vi "Averaged_Rot_Measure_Main_v1 Ś kopia.vi"() -> ()   [LabVIEW 2021]
uses:
  Config_File_Paths.ctl
  ZI_Data.ctl
  <vilib>/Utility/file.llb/Write Delimited Spreadsheet (DBL).vi
  <vilib>/measure/maspectr.llb/FFT Spectrum (Real-Im) for 1 Chan.vi
  <vilib>/Analysis/NI_AALPro.lvlib
  <vilib>/measure/NI_MAPro.lvlib
panel:
  out "single spectrum 2":waveform(dbl)[](graph)
  out "averaged spectrum":waveform(dbl)[](graph)
  out "single spectrum":waveform(dbl)[](graph)
  out "single differ":cluster{"Time":dbl[], "X":dbl[]}[](graph)
  out "single abs":cluster{"Time":dbl[], "X":dbl[]}[](graph)
  out "averaged rot":cluster{"Time":dbl[], "X":dbl[]}[](graph)
  out "single rot":cluster{"Time":dbl[], "X":dbl[]}[](graph)
  in  "Resource Address":T1={"ZI Address"="DEV714", "VISA Keithley"="", "VISA Arduino PG"=""}
  in  "error in":errorcluster
  in  "Config files paths":T2={"ZI config file (.ini)"="Config_Ver_1\\Zurich_params.ini", "Keithley config file (.ini)"="Config_Ver_1\\Keithley_params.ini", "Arduino config file (.ini)"="Config_Ver_1\\pulse_sequence.ini"}
  in  "Time unit":string(combo)="ms"
  out "loading":dbl(slide) scale=0.0..100.0
  in  "Number of averages":i32=1
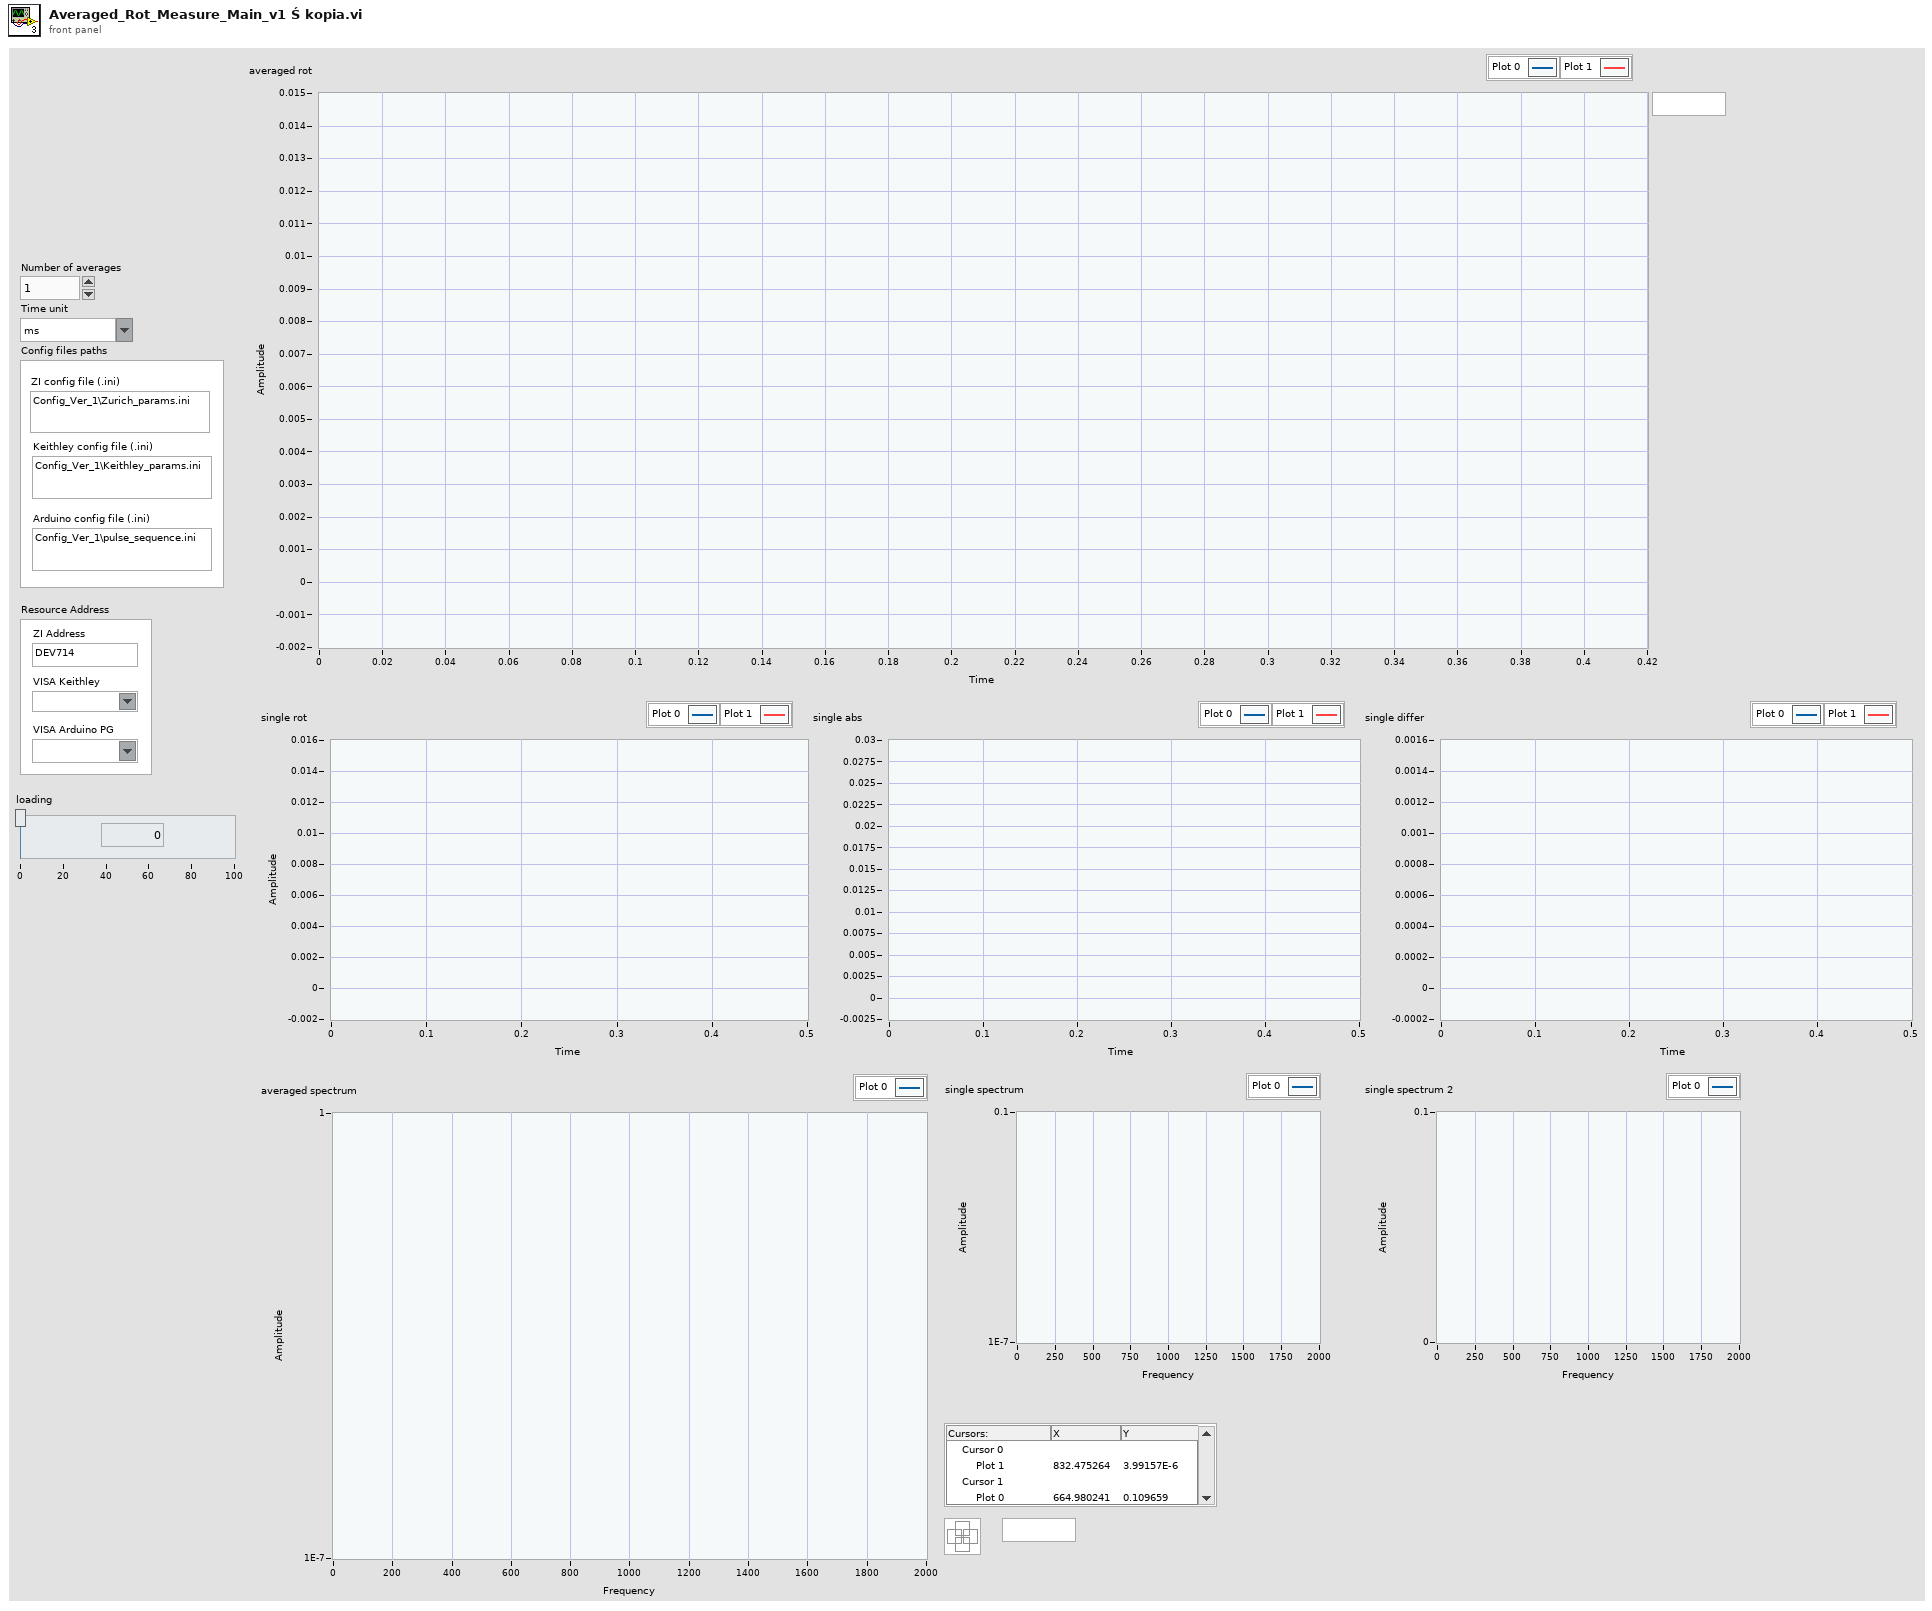
[diagram p1: front panel]
types:
  T1 = cluster{"ZI Address":string, "VISA Keithley":refnum<visa-resource-name>, "VISA Arduino PG":refnum<visa-resource-name>}
  T2 = typedef "Config_File_Paths.ctl" = cluster{"ZI config file (.ini)":string, "Keithley config file (.ini)":string, "Arduino config file (.ini)":string}
  T3 = typedef "ZI_Data.ctl" = cluster{"R":dbl[], "Theta":dbl[], "X":dbl[], "Y":dbl[], "AuxIn0":dbl[], "AuxIn1":dbl[], "Frequency":dbl[], "DIO":dbl[], "Time":dbl[]}
  T4 = typedef "Resources.ctl" = cluster{"ZI Handle":T5, "ZI ModHandle":T6, "VISA arduino":refnum<visa-resource-name>, "VISA Keithley":refnum<visa-resource-name>}
  T5 = typedef "Zurich Instruments LabOne.lvlib/ziTypeHandle.ctl" = cluster{"handleValid":bool, "Conn":u64, "Path Prefix":string, "Handle":u64, "Connected":bool, "Clockbase(s)":dbl}
  T6 = typedef "Zurich Instruments LabOne.lvlib/ziTypeModHandle.ctl" = cluster{"handleValid":bool, "Conn":u64, "ModHandle":u64, "moduleID":string, "Path Prefix":string}
  T7 = typedef "Cutted_Data.ctl" = cluster{"X":dbl[], "Y":dbl[], "Time":dbl[]}
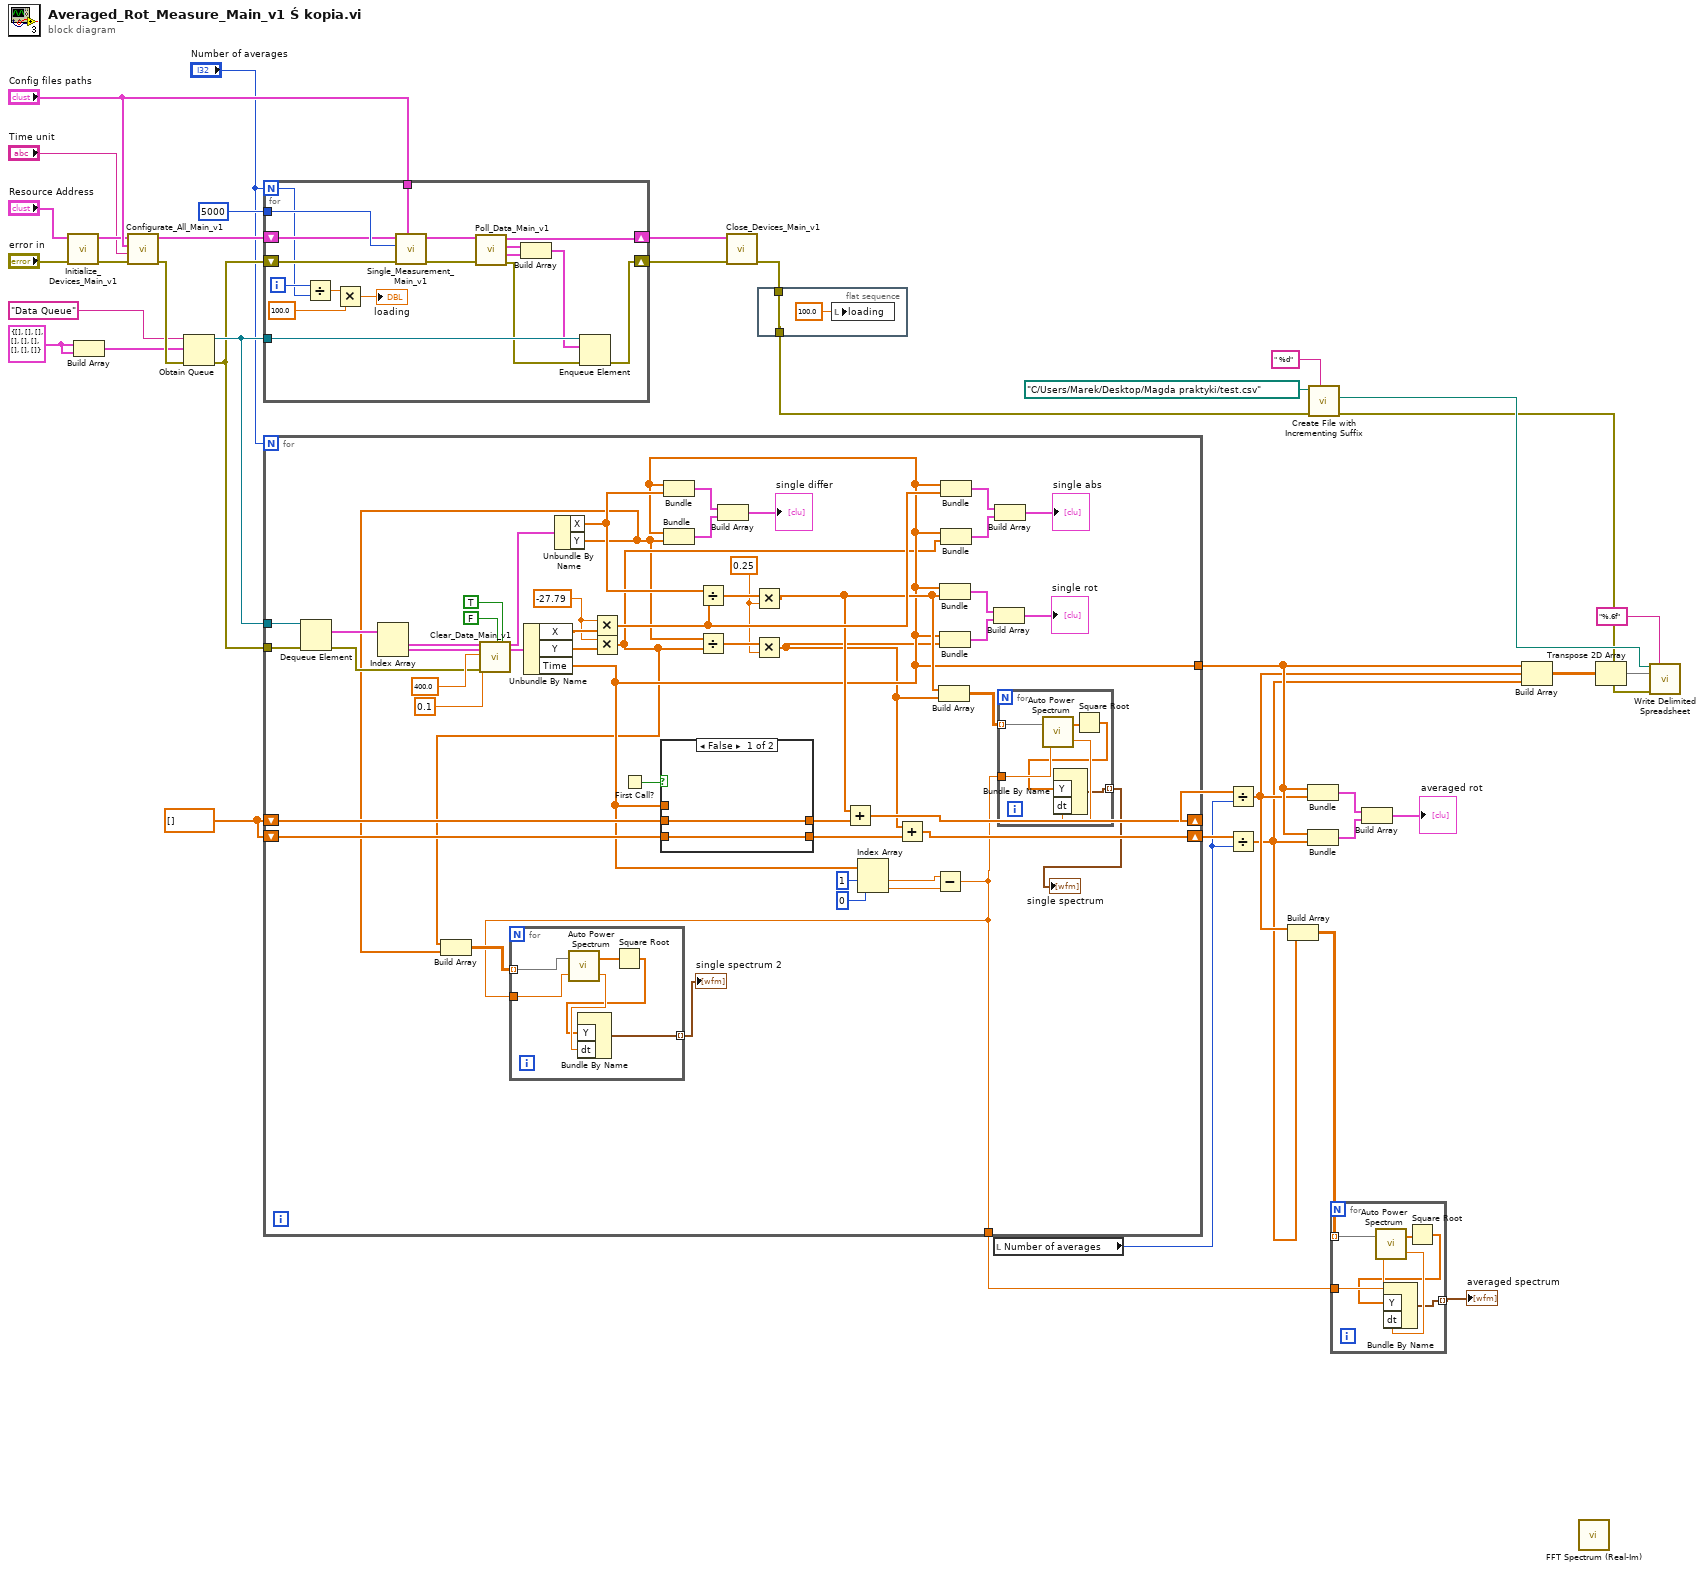
[diagram p0: block diagram]
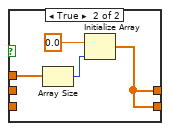
[diagram p2: hidden frame]
diagram:
  w23 = dbl[] []
  w27 = T3 {"R"=[], "Theta"=[], "X"=[], "Y"=[], "AuxIn0"=[], "AuxIn1"=[], "Frequency"=[], "DIO"=[], "Time"=[]} ("ZI Data")
  n1 = call "Initialize_Devices_Main_v1.vi"("error in"="error in", "Resource Address"="Resource Address") -> ("error out"=w31:errorcluster, "Resources"=w32:T4)  [unwired: 8 in]
  n2 = Build Array(w27, w27) -> (w26:T3[])
  n3 = call "Configurate_All_Main_v1.vi"("error in"=w31, "Time unit"="Time unit", "Config files paths"="Config files paths", "Resources in"=w32) -> ("error out"=w29:errorcluster, "Resources out"=w37:T4)  [unwired: 4 in, 2 out]
  n4 = Obtain Queue(name (unnamed)="Data Queue", element data type=w26, error in (no error)=w29) -> (queue out=w25:refnum<queue>, error out=w24:errorcluster)  [unwired: 2 in, 1 out]
  n5 = for {
    N: "Number of averages" -> [w49]
    shift-right: [w51] -> w38
    shift-left: w37 -> [w55]
    shift-right: [w40] -> w39
    shift-left: w24 -> [w54]
    tunnel: "Config files paths" -> [w57]
    tunnel: u64 5000 ("Timeout [ms]") -> [w56]
    tunnel: w25 -> [w45]
    i -> [w50]
    n6 = Divide(x=w50, y=w49) -> (x/y=w48:dbl)
    n7 = Multiply(x=w48, y=100.0) -> (x*y=→"loading":dbl)
    n8 = call "Single_Measurement_Main_v1.vi"("Config files paths"=w57, "error in"=w54, "Timeout [ms]"=w56, "Resources In"=w55) -> ("error out"=w52:errorcluster, "Resources Out"=w53:T4)  [unwired: 6 in]
    n9 = call "Poll_Data_Main_v1.vi"("error in"=w52, "Resources in"=w53) -> ("error out"=w41:errorcluster, "ZI Data 3"=w43:T3, "ZI Data 0"=w44:T3, "Resources out"=w51:T4)  [unwired: 6 in]
    n10 = Build Array(w44, w43) -> (w42:T3[])
    n11 = Enqueue Element(queue=w45, element=w42, error in (no error)=w41) -> (error out=w40:errorcluster)  [unwired: 1 in, 2 out]
  }
  n12 = for {
    N: "Number of averages" -> [_]
    tunnel: w25 -> [w107]
    tunnel: w24 -> [w106]
    shift-right: [w90] -> w20
    shift-left: w23 -> [w94]
    shift-right: [w89] -> w21
    shift-left: w23 -> [w93]
    tunnel: [w69] -> w9
    tunnel: [w58] -> w4
    w72 = 0.25
    w76 = -27.79
    n13 = Dequeue Element(queue=w107, error in (no error)=w106) -> (element=w105:T3[], error out=w100:errorcluster)  [unwired: 1 in, 2 out]
    n14 = Index Array(array=w105) -> (element #1=w104:T3, element #2=w103:T3)  [unwired: 2 in]
    n15 = call "Clear_Data_Main_v1.vi"("ZI Data 0"=w104, "ZI Data 3"=w103, "Time Of Collected Data (ms)"=400.0, "Crosstalk Tolerance"=0.1, "error in"=w100, "Fixed Number Of Points"=FALSE, "Check Phase Mismatch"=TRUE) -> ("Cutted Data"=w97:T7, "Cutted Data 3"=w96:T7)  [unwired: 7 in, 4 out]
    n16 = Unbundle By Name(w96) -> ("X"=w77:dbl[], "Y"=w78:dbl[], "Time"=w69:dbl[])
    n17 = Unbundle By Name(w97) -> ("X"=w79:dbl[], "Y"=w60:dbl[])
    n18 = Multiply(x=w76, y=w77) -> (x*y=w75:dbl[])
    n19 = Multiply(x=w76, y=w78) -> (x*y=w61:dbl[])
    n20 = Build Array(w61, w60) -> (w62:dbl[][])
    n21 = First Call?() -> (First Call?: T/F=w95:bool)
    n22 = case shown="False" w95 {
      tunnel: w69 -> [_ w125]
      tunnel: w94 -> [w121 _]
      tunnel: [w121 w122] -> w91
      tunnel: [w120 w122] -> w92
      tunnel: w93 -> [w120 _]
      frame False {
      }
      frame True {
        n23 = Array Size(array=w125) -> (size(s)=w123:i32)
        n24 = Initialize Array(0.0 ("element"), w123) -> (w122:dbl[])
      }
    }
    n25 = Bundle("Time"=w69, "X"=w79) -> (w82:cluster{"Time":dbl[], "X":dbl[]})  [unwired: 1 in]
    n26 = Bundle("Time"=w69, "Y"=w60) -> (w81:cluster{"Time":dbl[], "Y":dbl[]})  [unwired: 1 in]
    n27 = Divide(x=w79, y=w75) -> (x/y=w74:dbl[])
    n28 = Divide(x=w60, y=w61) -> (x/y=w73:dbl[])
    n29 = Build Array(w82, w81) -> (→"single differ":cluster{"Time":dbl[], "Y":dbl[]}[])
    n30 = Multiply(x=w74, y=w72) -> (x*y=w71:dbl[])
    n31 = Multiply(x=w73, y=w72) -> (x*y=w63:dbl[])
    n32 = Add(x=w71, y=w91) -> (x+y=w90:dbl[])
    n33 = Index Array(array=w69, index #1=1 ("index"), index #2=0 ("index")) -> (element #1=w66:dbl, element #2=w65:dbl)
    n34 = Add(x=w63, y=w92) -> (x+y=w89:dbl[])
    n35 = Subtract(x=w66, y=w65) -> (x-y=w58:dbl)
    n36 = for {
      tunnel: w62 -> [w113] mode=indexing
      tunnel: [w109] -> w59 mode=indexing
      tunnel: w58 -> [w108]
      n37 = call <vilib>:"Auto Power Spectrum.vi"("dt"=w108, "Signal (V)"=w113) -> ("df"=w112:dbl, "Power Spectrum (V^2 rms)"=w110:dbl[])
      n38 = Square Root(x=w110) -> (sqrt(x)=w111:dbl[])
      n39 = Bundle By Name("Y"=w111, "dt"=w112) -> (w109:waveform(dbl))  [unwired: 1 in]
    }
    "single spectrum 2" <- w59
    n40 = Build Array(w71, w63) -> (w70:dbl[][])
    n41 = Bundle("Time"=w69, w71) -> (w88:cluster{"Time":dbl[], dbl[]})  [unwired: 1 in]
    n42 = Bundle("Time"=w69, w63) -> (w87:cluster{"Time":dbl[], dbl[]})  [unwired: 1 in]
    n43 = Bundle("Time"=w69, w75) -> (w85:cluster{"Time":dbl[], dbl[]})  [unwired: 1 in]
    n44 = Bundle("Time"=w69, w61) -> (w84:cluster{"Time":dbl[], dbl[]})  [unwired: 1 in]
    n45 = Build Array(w88, w87) -> (→"single rot":cluster{"Time":dbl[], dbl[]}[])
    n46 = Build Array(w85, w84) -> (→"single abs":cluster{"Time":dbl[], dbl[]}[])
    n47 = for {
      tunnel: w70 -> [w119] mode=indexing
      tunnel: w58 -> [w118]
      tunnel: [w116] -> w64 mode=indexing
      n48 = call <vilib>:"Auto Power Spectrum.vi"("dt"=w118, "Signal (V)"=w119) -> ("df"=w117:dbl, "Power Spectrum (V^2 rms)"=w115:dbl[])
      n49 = Square Root(x=w115) -> (sqrt(x)=w114:dbl[])
      n50 = Bundle By Name("Y"=w114, "dt"=w117) -> (w116:waveform(dbl))  [unwired: 1 in]
    }
    "single spectrum" <- w64
  }
  n51 = call "Close_Devices_Main_v1.vi"("error in"=w39, "Resources in"=w38) -> ("error out"=w2:errorcluster)  [unwired: 9 in]
  n52 = flat-sequence {
    tunnel: [w126] -> w1
    tunnel: w2 -> [w126]
    frame #0 {
      n53 = local write "loading"(100.0 ("loading")) -> ()
    }
  }
  n54 = local read "Number of averages"() -> (w19:i32)
  n55 = Divide(x=w20, y=w19) -> (x/y=w7:dbl[])
  n56 = Divide(x=w21, y=w19) -> (x/y=w6:dbl[])
  n57 = Build Array(w7, w6) -> (w5:dbl[][])
  n58 = Bundle("Time"=w9, w7) -> (w16:cluster{"Time":dbl[], dbl[]})  [unwired: 1 in]
  n59 = Bundle("Time"=w9, w6) -> (w17:cluster{"Time":dbl[], dbl[]})  [unwired: 1 in]
  n60 = call <vilib>:"Create File with Incrementing Suffix.vi"("format string (\" (%d)\")"=" %d" ("format string (\" (%d)\")"), "error in (no error)"=w1, "file path"=path "C:/Users/Marek/Desktop/Magda praktyki/test.csv") -> ("error out"=w8:errorcluster, "actual path"=w10:path)  [unwired: 6 in, 1 out]
  n61 = for {
    tunnel: w5 -> [w133] mode=indexing
    tunnel: w4 -> [w132]
    tunnel: [w130] -> w3 mode=indexing
    n62 = call <vilib>:"Auto Power Spectrum.vi"("dt"=w132, "Signal (V)"=w133) -> ("df"=w131:dbl, "Power Spectrum (V^2 rms)"=w129:dbl[])
    n63 = Square Root(x=w129) -> (sqrt(x)=w128:dbl[])
    n64 = Bundle By Name("Y"=w128, "dt"=w131) -> (w130:waveform(dbl))  [unwired: 1 in]
  }
  "averaged spectrum" <- w3
  n65 = Build Array(w16, w17) -> (→"averaged rot":cluster{"Time":dbl[], dbl[]}[])
  n66 = Build Array(w9, w7, w6) -> (w13:dbl[][])
  n67 = call-poly <vilib>:"FFT Spectrum (Real-Im).vi"() -> ()  [unwired: 7 in, 5 out]
  n68 = Transpose 2D Array(2D array=w13) -> (transposed array=w12:dbl[][])
  n69 = call-poly <vilib>:"Write Delimited Spreadsheet.vi"("file path (dialog if empty)"=w10, "format (%.3f)"="%.6f", "2D data"=w12, "error in (no error)"=w8) -> ()  [unwired: 10 in, 2 out]
